vi "ECM.vi"() -> ()   [LabVIEW 2015]
panel:
  in  "Stop":bool
  out "Humidity":dbl(slide) scale=0.0..100.0
  out "Pressure":dbl(knob) scale=0.0..10.0
  out "Thermometer":dbl(slide) scale=0.0..100.0
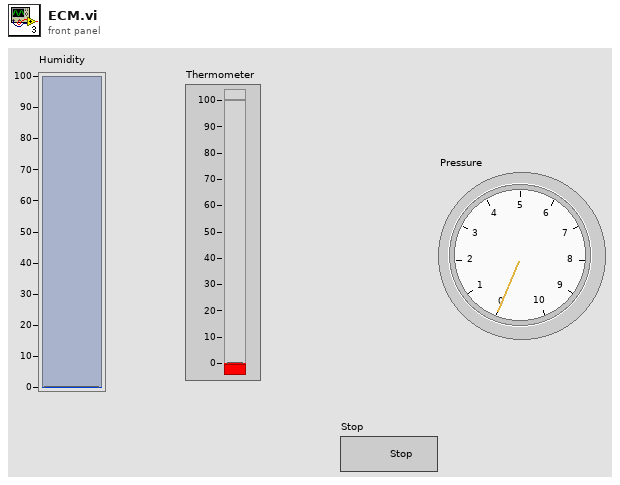
[diagram p1: front panel]
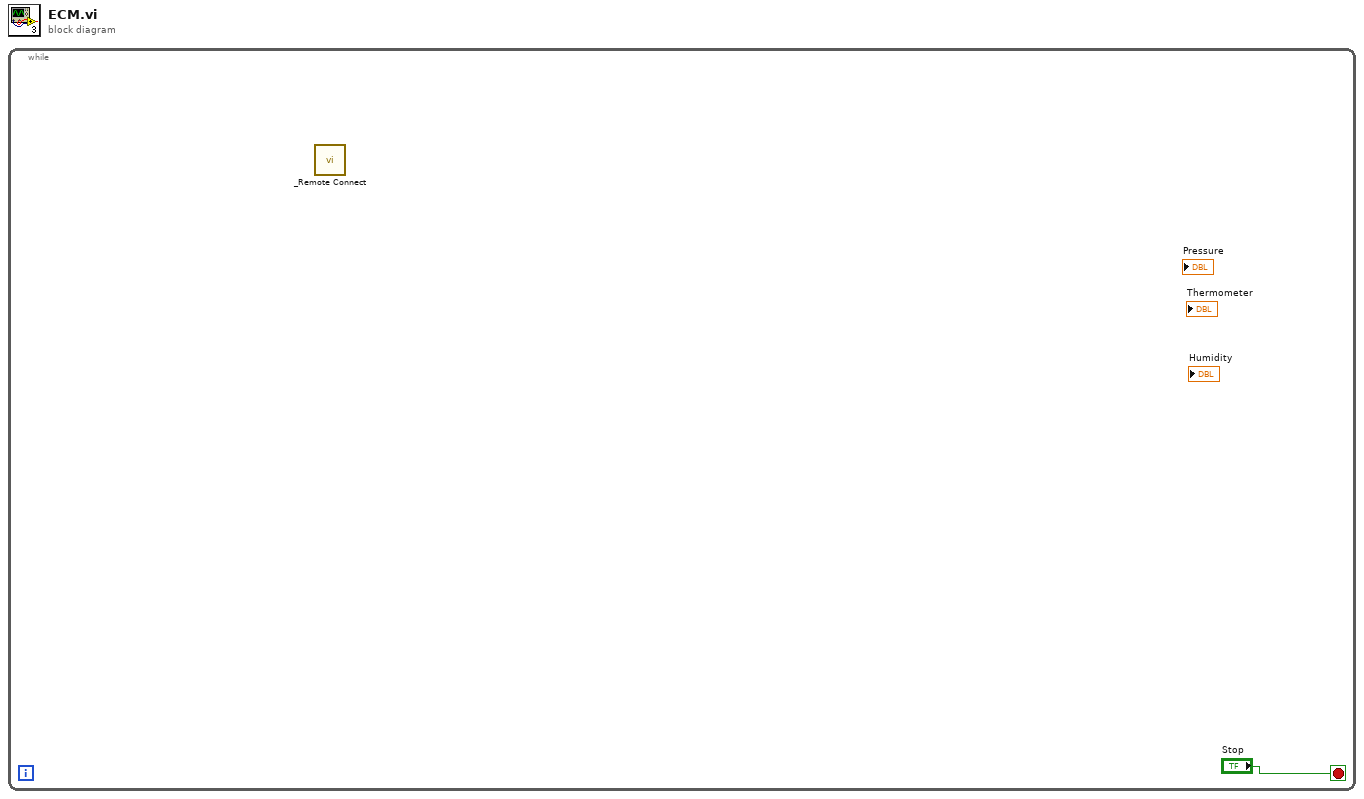
[diagram p0: block diagram]
diagram:
  n1 = while {
    stop <- "Stop" stop-if-true
    n2 = call "_Remote Connect.vi"() -> ()  [unwired: 6 in, 2 out]
  }
